vi "RemoveHiddenDevice.vi"(2 "error in (no error)":errorcluster, 3 "DeviceToShow":string, 4 "SetListPrefs in":refnum<class "SetListPrefs.lvclass">) -> (0 "error out":errorcluster, 1 "SetListPrefs out":refnum<class "SetListPrefs.lvclass">)   [LabVIEW 2013, in "SetListPrefs.lvclass"]
uses:
  SetListPrefs.lvclass
  SetListPrefs.lvclass/SetListPrefs.ctl
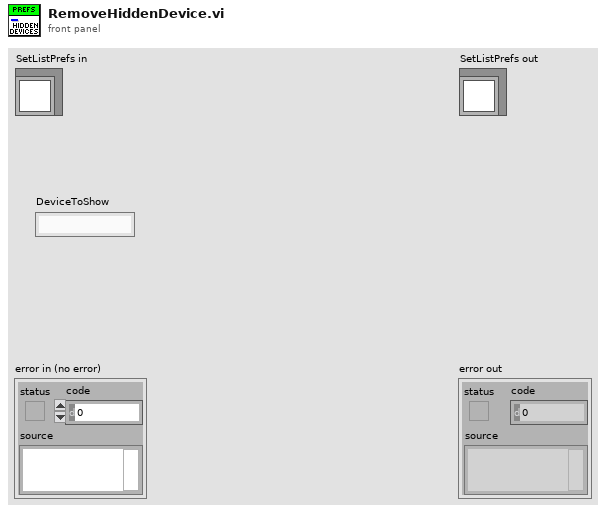
[diagram p1: front panel]
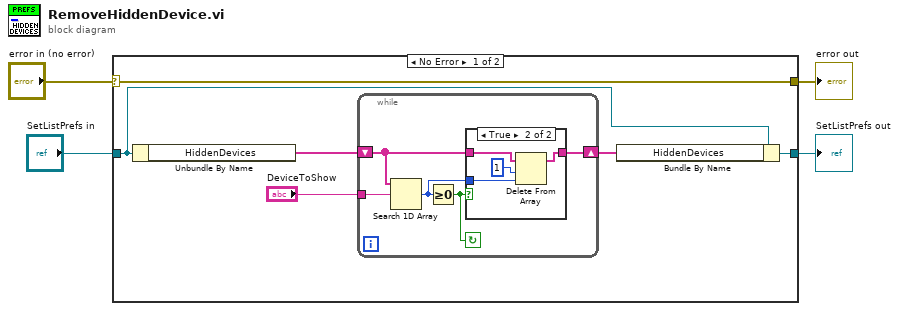
[diagram p0: block diagram]
diagram:
  n1 = case shown="No Error" "error in (no error)" {
    selector: "error in (no error)" -> [w10 w22]
    tunnel: [w10 w22] -> w3
    tunnel: [w8 w21] -> w1
    tunnel: "SetListPrefs in" -> [w9 w21]
    frame No Error {
      n2 = Unbundle By Name(w9) -> ("HiddenDevices"=w6:string[])
      n3 = while {
        tunnel: "DeviceToShow" -> [w15]
        shift-right: [w14] -> w5
        shift-left: w6 -> [w13]
        stop <- w11 continue-if-true
        n4 = Search 1D Array(1D array=w13, element=w15) -> (index of element=w12:i32)  [unwired: 1 in]
        n5 = Greater Or Equal To 0?(x=w12) -> (x >= 0?=w11:bool)
        n6 = case shown="True" w11 {
          tunnel: [w16 w19] -> w14
          tunnel: w13 -> [w16 w20]
          tunnel: w12 -> [_ w18]
          frame False {
          }
          frame True {
            n7 = Delete From Array(array=w20, length=1, index=w18) -> (array with subset deleted=w19:string[])  [unwired: 1 out]
          }
        }
      }
      n8 = Bundle By Name(cluster=w9, "HiddenDevices"=w5) -> (w8:refnum<class "SetListPrefs.lvclass">)
    }
    frame Error {
    }
  }
  "error out" <- w3
  "SetListPrefs out" <- w1
